vi "Initialize References.vi"(0 "Session Handle in":T2, 5 "References":T1, 11 "error in (no error)":errorcluster) -> (4 "Session Handle out":T2, 15 "error out":errorcluster)   [LabVIEW 2015, in "UI Handler.lvclass"]
uses:
  UI Handler.lvclass
  Typedefs/Session Handle.ctl
  Typedefs/References.ctl
  UI Handler.lvclass/UI Handler.ctl
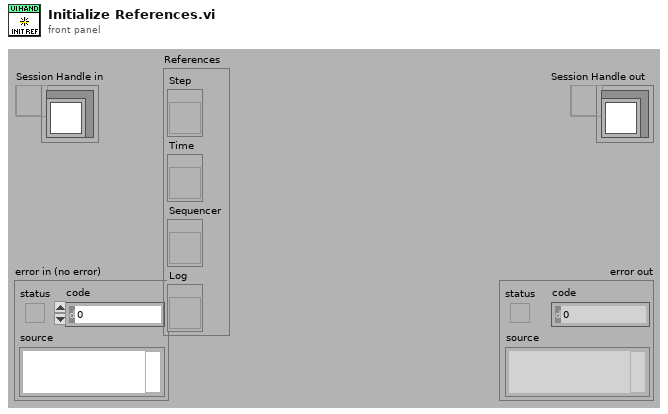
[diagram p1: front panel]
types:
  T1 = typedef "UI Handler.lvclass/References.ctl" = cluster{"Step":refnum<vi>, "Time":refnum<vi>, "Sequencer":refnum<vi>, "Log":refnum<vi>}
  T2 = typedef "UI Handler.lvclass/Session Handle.ctl" = refnum<data-value>
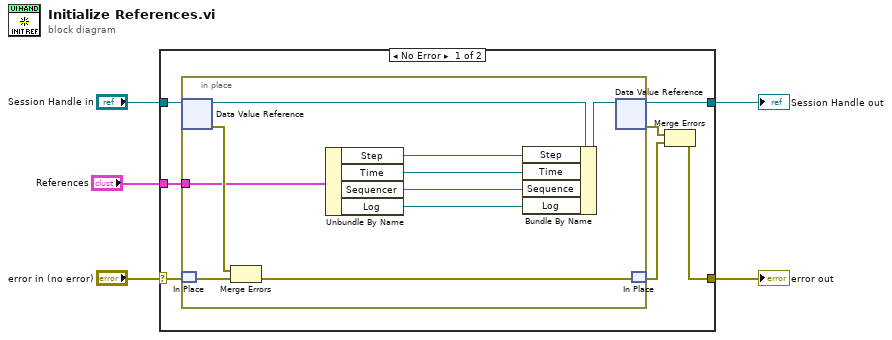
[diagram p0: block diagram]
diagram:
  n1 = case shown="No Error" "error in (no error)" {
    selector: "error in (no error)" -> [w7 w23]
    tunnel: "Session Handle in" -> [w12 w24]
    tunnel: [w11 w24] -> w4
    tunnel: [w8 w23] -> w3
    tunnel: "References" -> [w6 _]
    frame No Error {
      n2 = in-place {
        in-place-border: w6 -> [w17]
        n3 = in-place-dvr #1(w12) -> (w19:refnum<class "UI Handler.lvclass">, w21:errorcluster)
        n4 = in-place-match #2(w7) -> (w20:errorcluster)
        n5 = Merge Errors(w21, w20) -> (w22:errorcluster)
        n6 = Unbundle By Name(w17) -> ("Step"=w16:refnum<vi>, "Time"=w15:refnum<vi>, "Sequencer"=w14:refnum<vi>, "Log"=w13:refnum<vi>)
        n7 = Bundle By Name(cluster=w19, "Step"=w16, "Time"=w15, "Sequence"=w14, "Log"=w13) -> (w18:refnum<class "UI Handler.lvclass">)
        n8 = in-place-dvr #1(w18) -> (w11:T2, w9:errorcluster)
        n9 = in-place-match #2(w22) -> (w10:errorcluster)
      }
      n10 = Merge Errors(w9, w10) -> (w8:errorcluster)
    }
    frame Error {
    }
  }
  "Session Handle out" <- w4
  "error out" <- w3
